vi "Intsy_ResumeSerialStream.vi"() -> ()   [LabVIEW 2017]
panel:
  in  "StartSerialButton":bool
  out "DTscale for Serial Stream (s)":dbl
  out "error out":errorcluster
  in  "ADC_UART ratio":i16
  in  "ADC fs (Hz)":dbl
  out "Serial Port Type":string
  out "Teensy response":string
  in  "VISA resource name":refnum<visa-resource-name>="COM33"
  # "1. Choose COM port\n2. set ADC fs and ADC_UART ratio to indicator values shown  in main control panel\n3. Click Check in now"
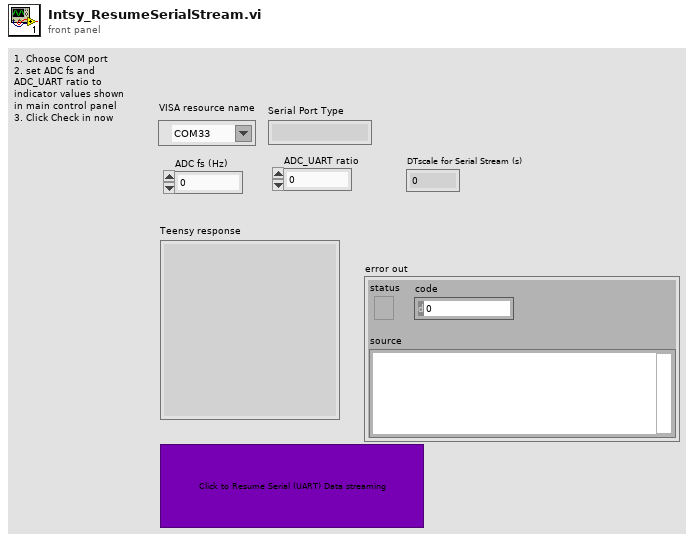
[diagram p1: front panel]
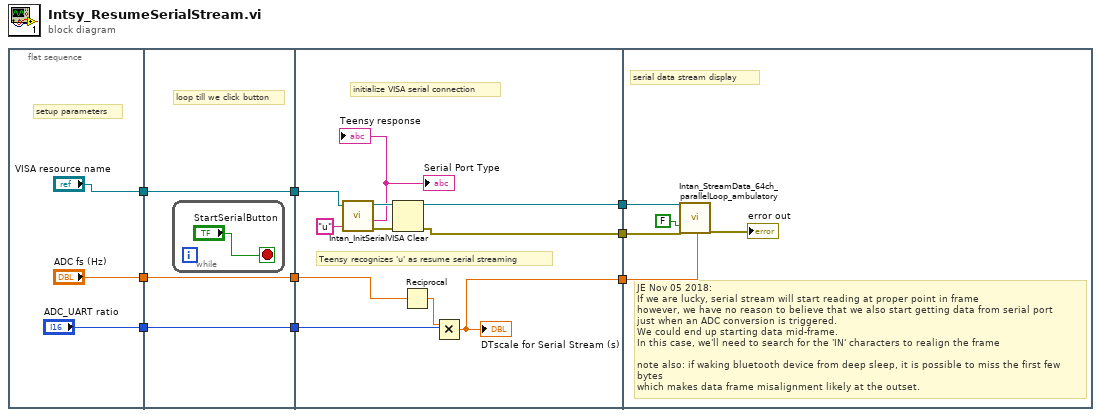
[diagram p0: block diagram]
diagram:
  n1 = flat-sequence {
    tunnel: ["VISA resource name"] -> w9
    tunnel: ["ADC fs (Hz)"] -> w7
    tunnel: ["ADC_UART ratio"] -> w5
    tunnel: w9 -> [w15]
    tunnel: [w15] -> w8
    tunnel: w7 -> [w14]
    tunnel: [w14] -> w6
    tunnel: w5 -> [w13]
    tunnel: [w13] -> w4
    tunnel: w8 -> [w27]
    tunnel: w6 -> [w23]
    tunnel: w4 -> [w21]
    tunnel: [w20] -> w3
    tunnel: [w19] -> w2
    tunnel: [w18] -> w1
    tunnel: w3 -> [w28]
    tunnel: w2 -> [w31]
    tunnel: w1 -> [w29]
    frame #0 {
      # "setup parameters"
    }
    frame #1 {
      # "loop till we click button"
      n2 = while {
        stop <- "StartSerialButton" stop-if-true
      }
    }
    frame #2 {
      # "Teensy recognizes 'u' as resume serial streaming"
      # "initialize VISA serial connection"
      n3 = call "Intan_InitSerial.vi"("VISA resource name"=w27, "InitialChar"="u") -> ("VISA resource name out"=w25:refnum<visa-resource-name>, "Text response"=→"Teensy response" →"Serial Port Type":string, "error out"=w26:errorcluster)  [unwired: 2 in]
      n4 = VISA Clear(VISA resource name=w25, error in (no error)=w26) -> (VISA resource name out=w19:refnum<visa-resource-name>, error out=w18:errorcluster)
      n5 = Reciprocal(x=w23) -> (1/x=w22:dbl)
      n6 = Multiply(x=w22, y=w21) -> (x*y=w20:dbl)
      "DTscale for Serial Stream (s)" <- w20
    }
    frame #3 {
      # "JE Nov 05 2018:\nIf we are lucky, serial stream will start reading at proper point in frame\nhowever, we have no reason to believe that we also start getting data from serial port\njust when an ADC conversion is triggered.\nWe could end up starting data mid-frame.  \nIn this case, we'll need to search for the 'IN' characters to realign the frame\n\nnote also: if waking bluetooth device from deep sleep, it is possible to miss the first few bytes\nwhich makes data frame misalignment likely at the outset."
      # "serial data stream display"
      n7 = call "Intan_StreamData_64ch_parallelLoop_ambulatory.vi"("VISA resource name"=w31, "Save Binary Data"=FALSE, "error in"=w29, "DT_scale (sec)"=w28) -> ("error out"=→"error out":errorcluster)  [unwired: 12 in, 3 out]
    }
  }
